vi "AndorInitCamera.vi"(8 "error in (no error)":errorcluster, 11 "Exposure":sgl) -> (0 "error out":errorcluster, 1 "accumulate out":sgl, 2 "exposure out":sgl, 3 "temperature out":sgl, 5 "kinetic out":sgl)   [LabVIEW 2018, in "AndorOWN.lvlib"]
uses:
  AndorOWN.lvlib
  Andor SDK/AndorSDK.lvlib
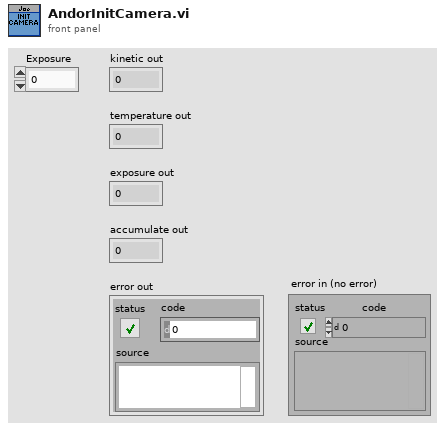
[diagram p1: front panel]
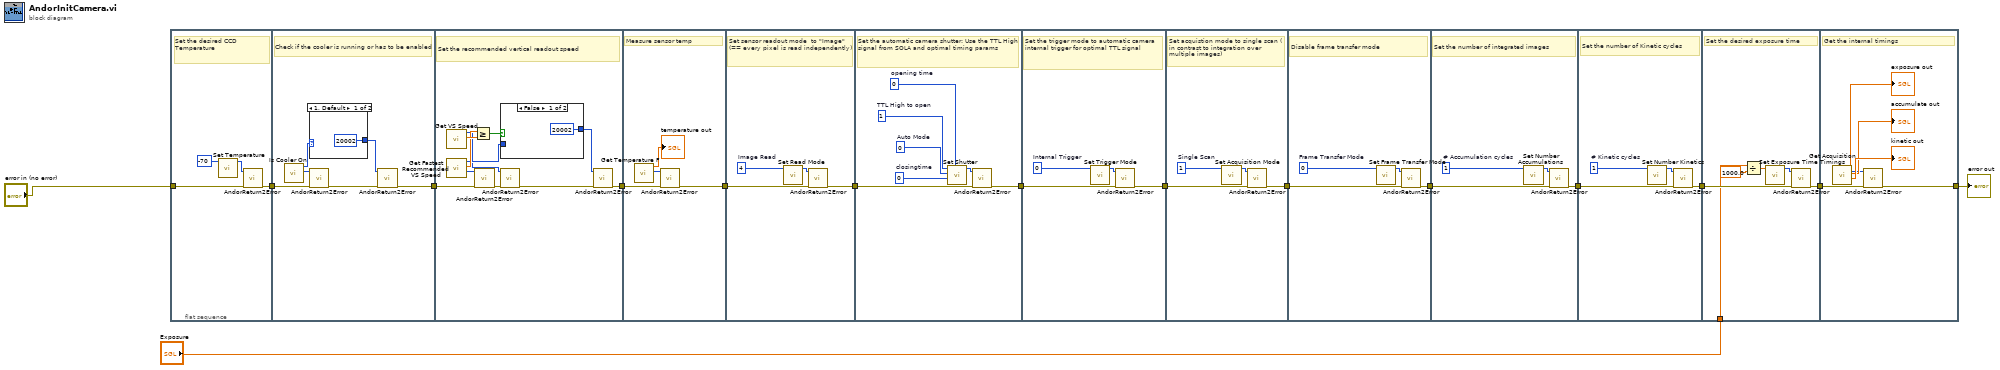
[diagram p0: block diagram]
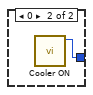
[diagram p2: hidden frame]
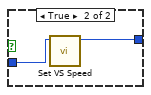
[diagram p3: hidden frame]
diagram:
  n1 = flat-sequence {
    tunnel: [w17] -> w2
    tunnel: "error in (no error)" -> [w16]
    tunnel: [w23] -> w15
    tunnel: w2 -> [w20]
    tunnel: w15 -> [w34]
    tunnel: [w32] -> w14
    tunnel: w14 -> [w45]
    tunnel: [w44] -> w13
    tunnel: w13 -> [w48]
    tunnel: [w47] -> w12
    tunnel: w12 -> [w51]
    tunnel: [w52] -> w11
    tunnel: w11 -> [w59]
    tunnel: [w58] -> w10
    tunnel: w10 -> [w63]
    tunnel: [w62] -> w9
    tunnel: w9 -> [w67]
    tunnel: [w66] -> w8
    tunnel: w8 -> [w71]
    tunnel: [w69] -> w7
    tunnel: w7 -> [w76]
    tunnel: [w75] -> w6
    tunnel: w6 -> [w80]
    tunnel: "Exposure" -> [w78]
    tunnel: [w77] -> w4
    tunnel: w4 -> [w84]
    tunnel: [w83] -> w3
    frame #0 {
      # "Set the desired CCD Temperature"
      n2 = call "Set Temperature.vi"("temperature"=-70) -> ("function return"=w18:u32)  [unwired: 9 in, 1 out]
      n3 = call "AndorReturn2Error.vi"("error in (no error)"=w16, "Camera return"=w18) -> ("error out"=w17:errorcluster)  [unwired: 9 in]
    }
    frame #1 {
      # "Check if the cooler is running or has to be enabled"
      n4 = call "Is Cooler On.vi"() -> ("function return"=w22:u32, "iCoolerStatus out"=w25:i32)  [unwired: 9 in, 1 out]
      n5 = case shown="1, Default" w25 {
        tunnel: [u32 20002 ("function return") w27] -> w21
        frame 1, Default {
        }
        frame 0 {
          n6 = call "Cooler ON.vi"() -> ("function return"=w27:u32)  [unwired: 10 in, 1 out]
        }
      }
      n7 = call "AndorReturn2Error.vi"("error in (no error)"=w20, "Camera return"=w22) -> ("error out"=w24:errorcluster)  [unwired: 9 in]
      n8 = call "AndorReturn2Error.vi"("error in (no error)"=w24, "Camera return"=w21) -> ("error out"=w23:errorcluster)  [unwired: 9 in]
    }
    frame #2 {
      # "Set the recommended vertical readout speed"
      n9 = call "Get VS Speed.vi"() -> ("speed out"=w38:sgl, "function return"=w29:u32)  [unwired: 9 in, 1 out]
      n10 = call "Get Fastest Recommended VS Speed.vi"() -> ("function return"=w30:u32, "speed out"=w37:sgl, "index out"=w35:i32)  [unwired: 8 in, 1 out]
      n11 = Greater Or Equal?(x=w37, y=w38) -> (x >= y?=w36:bool)
      n12 = call "AndorReturn2Error.vi"("error in (no error)"=w34, "Camera return"=w30) -> ("error out"=w33:errorcluster)  [unwired: 9 in]
      n13 = case shown="False" w36 {
        tunnel: w35 -> [_ w41]
        tunnel: [u32 20002 ("function return") w40] -> w28
        frame False {
        }
        frame True {
          n14 = call "Set VS Speed.vi"("index"=w41) -> ("function return"=w40:u32)  [unwired: 10 in]
        }
      }
      n15 = call "AndorReturn2Error.vi"("error in (no error)"=w33, "Camera return"=w29) -> ("error out"=w31:errorcluster)  [unwired: 9 in]
      n16 = call "AndorReturn2Error.vi"("error in (no error)"=w31, "Camera return"=w28) -> ("error out"=w32:errorcluster)  [unwired: 9 in]
    }
    frame #3 {
      # "Measure sensor temp"
      n17 = call "Get Temperature F.vi"() -> ("function return"=w42:u32, "temperature out"=→"temperature out":sgl)  [unwired: 9 in, 1 out]
      n18 = call "AndorReturn2Error.vi"("error in (no error)"=w45, "Camera return"=w42) -> ("error out"=w44:errorcluster)  [unwired: 9 in]
    }
    frame #4 {
      w49 = 4  # Image Read
      # "Set sensor readout mode  to \"Image\" (== every pixel is read independently)"
      n19 = call "Set Read Mode.vi"("mode"=w49) -> ("function return"=w46:u32)  [unwired: 9 in, 1 out]
      n20 = call "AndorReturn2Error.vi"("error in (no error)"=w48, "Camera return"=w46) -> ("error out"=w47:errorcluster)  [unwired: 9 in]
    }
    frame #5 {
      w56 = 0  # opening time
      w54 = 0  # Auto Mode
      w53 = 1  # TTL High to open
      w55 = 0  # closingtime
      # "Set the automatic camera shutter: Use the TTL High signal from SOLA and optimal timing params"
      n21 = call "Set Shutter.vi"("openingtime"=w56, "closingtime"=w55, "mode"=w54, "typ"=w53) -> ("function return"=w50:u32)  [unwired: 6 in, 1 out]
      n22 = call "AndorReturn2Error.vi"("error in (no error)"=w51, "Camera return"=w50) -> ("error out"=w52:errorcluster)  [unwired: 9 in]
    }
    frame #6 {
      w60 = 0  # Internal Trigger
      # "Set the trigger mode to automatic camera internal trigger for optimal TTL signal"
      n23 = call "Set Trigger Mode.vi"("mode"=w60) -> ("function return"=w57:u32)  [unwired: 9 in, 1 out]
      n24 = call "AndorReturn2Error.vi"("error in (no error)"=w59, "Camera return"=w57) -> ("error out"=w58:errorcluster)  [unwired: 9 in]
    }
    frame #7 {
      w64 = 1  # Single Scan
      # "Set acquistion mode to single scan ( in contrast to integration over multiple images)"
      n25 = call "Set Acquisition Mode.vi"("mode"=w64) -> ("function return"=w61:u32)  [unwired: 9 in, 1 out]
      n26 = call "AndorReturn2Error.vi"("error in (no error)"=w63, "Camera return"=w61) -> ("error out"=w62:errorcluster)  [unwired: 9 in]
    }
    frame #8 {
      w68 = 0  # Frame Transfer Mode
      # "Disable frame transfer mode"
      n27 = call "Set Frame Transfer Mode.vi"("mode"=w68) -> ("function return"=w65:u32)  [unwired: 10 in]
      n28 = call "AndorReturn2Error.vi"("error in (no error)"=w67, "Camera return"=w65) -> ("error out"=w66:errorcluster)  [unwired: 9 in]
    }
    frame #9 {
      w70 = 1  # # Accumulation cycles
      # "Set the number of integrated images"
      n29 = call "Set Number Accumulations.vi"("number"=w70) -> ("function return"=w72:u32)  [unwired: 9 in, 1 out]
      n30 = call "AndorReturn2Error.vi"("error in (no error)"=w71, "Camera return"=w72) -> ("error out"=w69:errorcluster)  [unwired: 9 in]
    }
    frame #10 {
      w74 = 1  # # Kinetic cycles
      # "Set the number of Kinetic cycles"
      n31 = call "Set Number Kinetics.vi"("number"=w74) -> ("function return"=w73:u32)  [unwired: 9 in, 1 out]
      n32 = call "AndorReturn2Error.vi"("error in (no error)"=w76, "Camera return"=w73) -> ("error out"=w75:errorcluster)  [unwired: 9 in]
    }
    frame #11 {
      # "Set the desired exposure time"
      n33 = Divide(x=w78, y=sgl 1000.0) -> (x/y=w82:sgl)
      n34 = call "Set Exposure Time.vi"("time"=w82) -> ("function return"=w81:u32)  [unwired: 9 in, 1 out]
      n35 = call "AndorReturn2Error.vi"("error in (no error)"=w80, "Camera return"=w81) -> ("error out"=w77:errorcluster)  [unwired: 9 in]
    }
    frame #12 {
      # "Get the internal timings"
      n36 = call "Get Acquisition Timings.vi"() -> ("kinetic out"=→"kinetic out":sgl, "accumulate out"=→"accumulate out":sgl, "exposure out"=→"exposure out":sgl, "function return"=w85:u32)  [unwired: 7 in, 1 out]
      n37 = call "AndorReturn2Error.vi"("error in (no error)"=w84, "Camera return"=w85) -> ("error out"=w83:errorcluster)  [unwired: 9 in]
    }
  }
  "error out" <- w3
